vi "ReadOldCarexFile.vi"(6 "error in (no error)":errorcluster, 8 "OldCarexFilePath":path, 9 "CarexData In":refnum<class "CarexMData.lvclass">) -> (0 "error out":errorcluster, 1 "all rows":dbl[][](array[numeric]) format="%0.3f", 3 "CarexData Out":refnum<class "CarexMData.lvclass">)   [LabVIEW 2014]
uses:
  <vilib>/Utility/file.llb/Read From Spreadsheet File (DBL).vi
  <vilib>/Utility/miscctls.llb/LVDateTimeRec.ctl
  CarexMData.lvclass
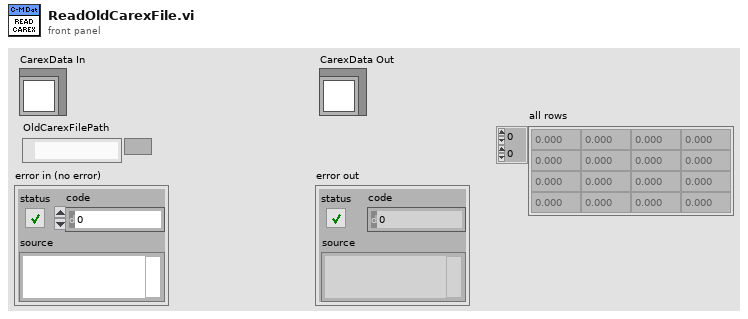
[diagram p1: front panel]
types:
  T1 = cluster{"MotorOn":bool, "EstGH":bool, "TensionMode":u16}
  T2 = typedef "LVDateTimeRec.ctl" = cluster{"fractional second":dbl, "second":i32, "minute":i32, "hour":i32, "day of month":i32, "month":i32, "year":i32, "day of week":i32, "day of year":i32, "DST":i32}
  T3 = cluster{"array type (2D Dbl)[0]":dbl, "array type (2D Dbl)[1]":dbl}
  T4 = cluster{"array type (2D Dbl)[0]":dbl, "array type (2D Dbl)[1]":dbl, "array type (2D Dbl)[2]":dbl, "array type (2D Dbl)[3]":dbl, "array type (2D Dbl)[4]":dbl, "array type (2D Dbl)[5]":dbl}
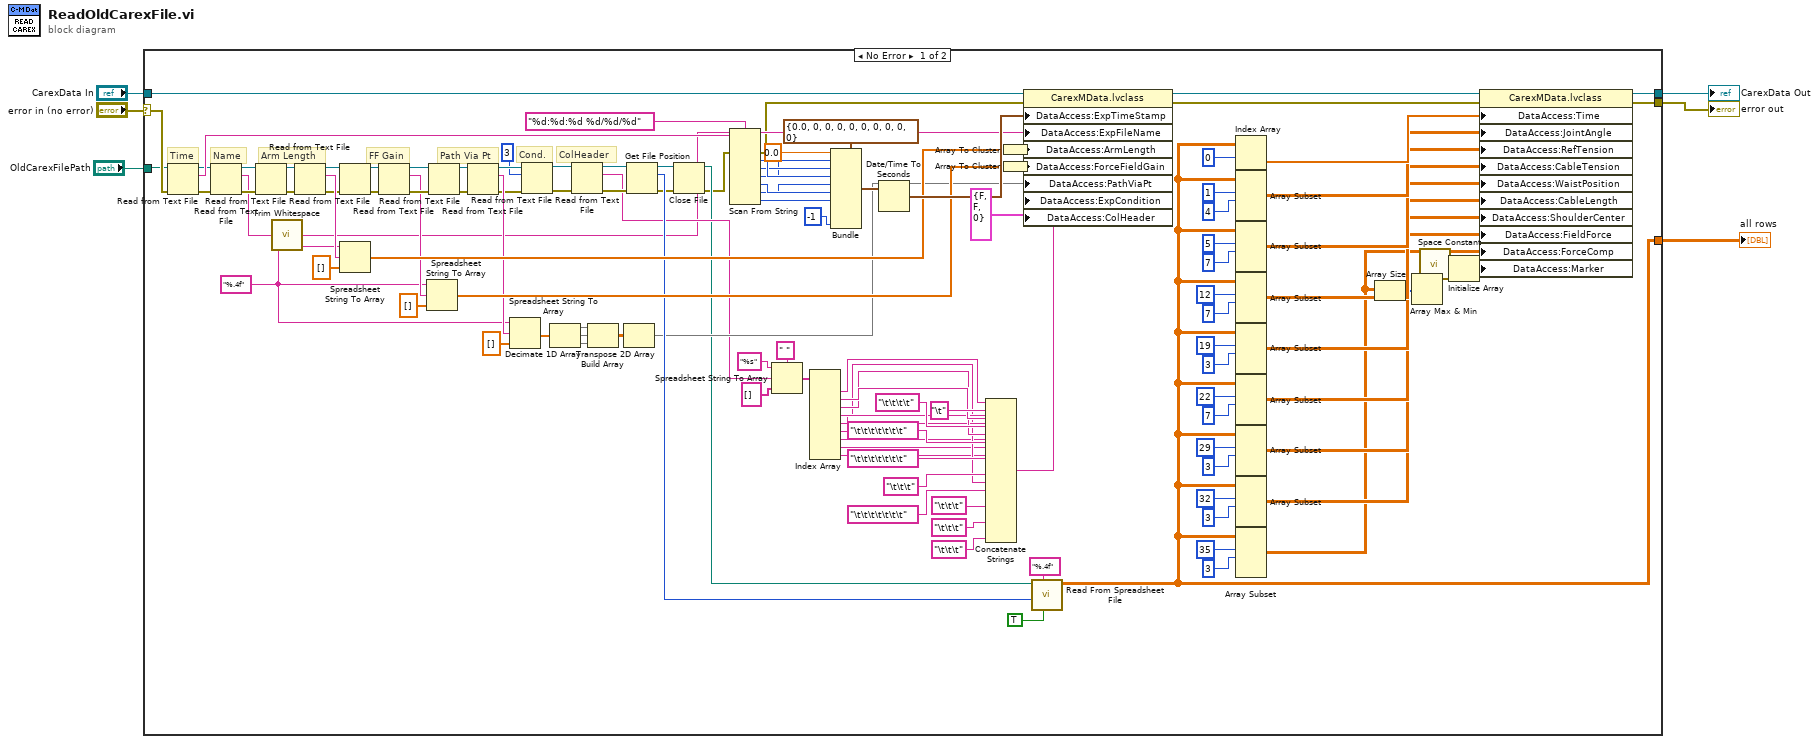
[diagram p0: block diagram]
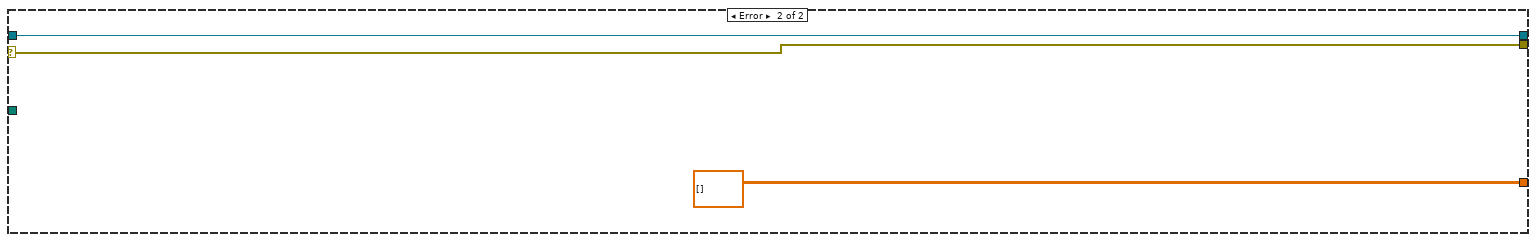
[diagram p2: hidden frame]
diagram:
  n1 = case shown="No Error" "error in (no error)" {
    selector: "error in (no error)" -> [w84 w133]
    tunnel: "OldCarexFilePath" -> [w54 _]
    tunnel: [w17 dbl[][] [] ("all rows")] -> w5
    tunnel: "CarexData In" -> [w112 w132]
    tunnel: [w129 w132] -> w2
    tunnel: [w110 w133] -> w1
    frame No Error {
      w55 = "%.4f" ("format (%.3f)")
      # "ColHeader"
      # "Cond."
      # "Path Via Pt"
      # "FF Gain"
      # "Arm Length"
      # "Name"
      # "Time"
      n2 = Read from Text File(file (use dialog)=w54, error in=w84) -> (refnum out=w86:refnum<file>, text=w87:string, error out=w85:errorcluster)  [unwired: 2 in, 1 out]
      n3 = Read from Text File(file (use dialog)=w86, error in=w85) -> (refnum out=w83:refnum<file>, text=w20:string, error out=w82:errorcluster)  [unwired: 2 in, 1 out]
      n4 = Read from Text File(file (use dialog)=w83, error in=w82) -> (refnum out=w81:refnum<file>, error out=w80:errorcluster)  [unwired: 2 in, 2 out]
      n5 = call <vilib>:"Trim Whitespace.vi"("string"=w20) -> ("trimmed string"=w19:string)  [unwired: 1 in]
      n6 = Read from Text File(file (use dialog)=w81, error in=w80) -> (refnum out=w74:refnum<file>, text=w79:string, error out=w75:errorcluster)  [unwired: 2 in, 1 out]
      n7 = Read from Text File(file (use dialog)=w74, error in=w75) -> (refnum out=w72:refnum<file>, error out=w73:errorcluster)  [unwired: 2 in, 2 out]
      n8 = Spreadsheet String To Array(format string=w55, spreadsheet string=w79, array type (2D Dbl)=dbl[] []) -> (array=w77:dbl[])  [unwired: 1 in]
      n9 = Read from Text File(file (use dialog)=w72, error in=w73) -> (refnum out=w66:refnum<file>, text=w56:string, error out=w65:errorcluster)  [unwired: 2 in, 1 out]
      n10 = Spreadsheet String To Array(format string=w55, spreadsheet string=w56, array type (2D Dbl)=dbl[] []) -> (array=w69:dbl[])  [unwired: 1 in]
      n11 = Read from Text File(file (use dialog)=w66, error in=w65) -> (refnum out=w68:refnum<file>, error out=w67:errorcluster)  [unwired: 2 in, 2 out]
      n12 = Read from Text File(file (use dialog)=w68, error in=w67) -> (refnum out=w53:refnum<file>, text=w63:string, error out=w52:errorcluster)  [unwired: 2 in, 1 out]
      n13 = Spreadsheet String To Array(format string=w55, spreadsheet string=w63, array type (2D Dbl)=dbl[] []) -> (array=w62:dbl[])  [unwired: 1 in]
      n14 = Read from Text File(file (use dialog)=w53, count=3, error in=w52) -> (refnum out=w45:refnum<file>, error out=w46:errorcluster)  [unwired: 1 in, 2 out]
      n15 = Decimate 1D Array(w62) -> (w61:dbl[], w60:dbl[], w59:dbl[])
      n16 = Read from Text File(file (use dialog)=w45, error in=w46) -> (refnum out=w47:refnum<file>, text=w44:string, error out=w48:errorcluster)  [unwired: 2 in, 1 out]
      n17 = Build Array(w61, w60, w59) -> (w58:dbl[][])
      n18 = Transpose 2D Array(2D array=w58) -> (transposed array=w49:dbl[][])
      n19 = Get File Position(4:w48, 7:w47) -> (0:w10:errorcluster, 2:w50:i64, 3:w9:refnum<file>)
      n20 = Close File(refnum=w9, error in=w10) -> (path=w8:path, error out=w7:errorcluster)
      n21 = Scan From String(format string="%d:%d:%d %d/%d/%d", input string=w87, error in=w7) -> (error out=w18:errorcluster, output 1=w95:i32, output 2=w94:i32, output 3=w93:i32, output 4=w92:i32, output 5=w91:i32, output 6=w90:i32)  [unwired: 7 in, 2 out]
      n22 = Spreadsheet String To Array(delimiter (Tab)=" ", format string="%s", spreadsheet string=w44, array type (2D Dbl)=string[] []) -> (array=w40:string[])
      n23 = Index Array(array=w40) -> (element #1=w39:string, element #2=w37:string, element #3=w35:string, element #4=w33:string, element #5=w31:string, element #6=w29:string, element #7=w27:string, element #8=w25:string, element #9=w23:string)  [unwired: 9 in]
      n24 = Bundle(cluster=T2 {"fractional second"=0.0, "second"=0, "minute"=0, "hour"=0, "day of month"=0, "month"=0, "year"=0, "day of week"=0, "day of year"=0, "DST"=0} ("date time rec"), "fractional second"=0.0, "second"=w93, "minute"=w94, "hour"=w95, "day of month"=w91, "month"=w92, "year"=w90, "DST"=-1) -> (w96:T2)  [unwired: 2 in]
      n25 = Date/Time To Seconds(2:w96) -> (0:w89:timestamp)  [unwired: 1 in]
      n26 = Concatenate Strings(w39, "\t" ("delimiter (Tab)"), w37, "\t\t\t\t" ("delimiter (Tab)"), w35, "\t\t\t\t\t\t\t" ("delimiter (Tab)"), w33, "\t\t\t\t\t\t\t" ("delimiter (Tab)"), w31, "\t\t\t" ("delimiter (Tab)"), w29, "\t\t\t\t\t\t\t" ("delimiter (Tab)"), w27, "\t\t\t" ("delimiter (Tab)"), w25, "\t\t\t" ("delimiter (Tab)"), w23, "\t\t\t" ("delimiter (Tab)")) -> (w21:string)
      n27 = Array To Cluster(array=w77) -> (cluster=w78:T3)
      n28 = Array To Cluster(array=w69) -> (cluster=w70:T4)
      n29 = property class="CarexMData.lvclass"(reference=w112, error in=w18, "DataAccess:ExpTimeStamp"=w89, "DataAccess:ExpFileName"=w19, "DataAccess:ArmLength"=w78, "DataAccess:ForceFieldGain"=w70, "DataAccess:PathViaPt"=w49, "DataAccess:ExpCondition"=T1 {"MotorOn"=FALSE, "EstGH"=FALSE, "TensionMode"=0} ("ExpCondition"), "DataAccess:ColHeader"=w21) -> (reference out=w113:refnum<class "CarexMData.lvclass">, error out=w111:errorcluster)
      n30 = call-poly <vilib>:"Read From Spreadsheet File.vi"("transpose (no:F)"=TRUE, "format (%.3f)"="%.4f", "start of read offset (chars.:0)"=w50, "file path (dialog if empty)"=w8) -> ("all rows"=w17:dbl[][])  [unwired: 3 in, 4 out]
      n31 = Index Array(array=w17, index (row)=0 ("index")) -> (element=w109:dbl[])  [unwired: 1 in]
      n32 = Array Subset(array=w17, index (row)=1 ("index"), length (row)=4 ("length")) -> (w108:dbl[][])  [unwired: 2 in]
      n33 = Array Subset(array=w17, index (row)=5 ("index"), length (row)=7 ("length")) -> (w107:dbl[][])  [unwired: 2 in]
      n34 = Array Subset(array=w17, index (row)=12 ("index"), length (row)=7 ("length")) -> (w106:dbl[][])  [unwired: 2 in]
      n35 = Array Subset(array=w17, index (row)=19 ("index"), length (row)=3 ("length")) -> (w105:dbl[][])  [unwired: 2 in]
      n36 = Array Subset(array=w17, index (row)=22 ("index"), length (row)=7 ("length")) -> (w104:dbl[][])  [unwired: 2 in]
      n37 = Array Subset(array=w17, index (row)=29 ("index"), length (row)=3 ("length")) -> (w103:dbl[][])  [unwired: 2 in]
      n38 = Array Subset(array=w17, index (row)=32 ("index"), length (row)=3 ("length")) -> (w100:dbl[][])  [unwired: 2 in]
      n39 = Array Subset(array=w17, index (row)=35 ("index"), length (row)=3 ("length")) -> (w15:dbl[][])  [unwired: 2 in]
      n40 = Array Size(array=w15) -> (size(s)=w14:i32[])
      n41 = Array Max & Min(array=w14) -> (max value=w11:i32)  [unwired: 3 out]
      n42 = call <vilib>:"Space Constant.vi"() -> ("String"=w12:string)
      n43 = Initialize Array(w12, w11) -> (w13:string[])
      n44 = property class="CarexMData.lvclass"(reference=w113, error in=w111, "DataAccess:Time"=w109, "DataAccess:JointAngle"=w108, "DataAccess:RefTension"=w107, "DataAccess:CableTension"=w106, "DataAccess:WaistPosition"=w105, "DataAccess:CableLength"=w104, "DataAccess:ShoulderCenter"=w103, "DataAccess:FieldForce"=w100, "DataAccess:ForceComp"=w15, "DataAccess:Marker"=w13) -> (reference out=w129:refnum<class "CarexMData.lvclass">, error out=w110:errorcluster)
    }
    frame Error {
    }
  }
  "all rows" <- w5
  "CarexData Out" <- w2
  "error out" <- w1
